vi "Get Vector - stdout.vi"(6 "no transpose\nfor reading":bool, 8 "error in (no error)":errorcluster, 9 "octave vector sizes":i32[](array[numeric]), 10 "variable name":string, 11 "pipe in":T1) -> (0 "error out":errorcluster, 2 "vector":string[](array[string]), 3 "pipe out":T1, 4 "value transposed?":bool)   [LabVIEW 2013, in "GOLPI library.lvlib"]
doc: "Reads vector variable from GNU Octave. Returns output as array of strings. Internaly converts row vector to column for simpler parsing of long vectors. It means complex vectors are conjugated and strings are incorrectly parsed. If 'no transpose for reading' is set true, function reads row vectors as rows."
uses:
  GOLPI library.lvlib
  LV Process.lvlibp/Pipe Handle.ctl
  Custom Error Codes Enum Type Def.vi
  Globals.vi
  LV Process.lvlibp
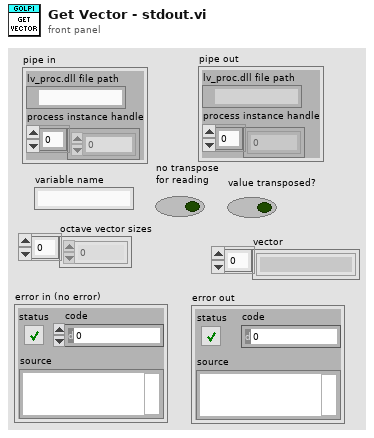
[diagram p1: front panel]
types:
  T1 = typedef "LV Process.lvlibp/Pipe Handle.ctl" = cluster{"lv_proc.dll file path":path, "process instance handle":u32[]}
  T2 = typedef "GOLPI library.lvlib/Custom Error Codes Enum Type Def.vi" = enum16{"no error", "00 working directory PAR1 missing", "01 octave binary PAR1 missing", "02 octave report error PAR1", "03 empty output last cmd PAR1", "04 missing temporary file PAR1", "10 var PAR1 not string", "11 var PAR1 not num, scal, ~compl", "12 var PAR1 not num, scal, compl", "13 var PAR1 not num, vect, ~compl", "14 var PAR1 not num, vect, compl", "15 var PAR1 not num, mat, ~compl", "16 var PAR1 not num, mat, ~compl", "99 not finished"}
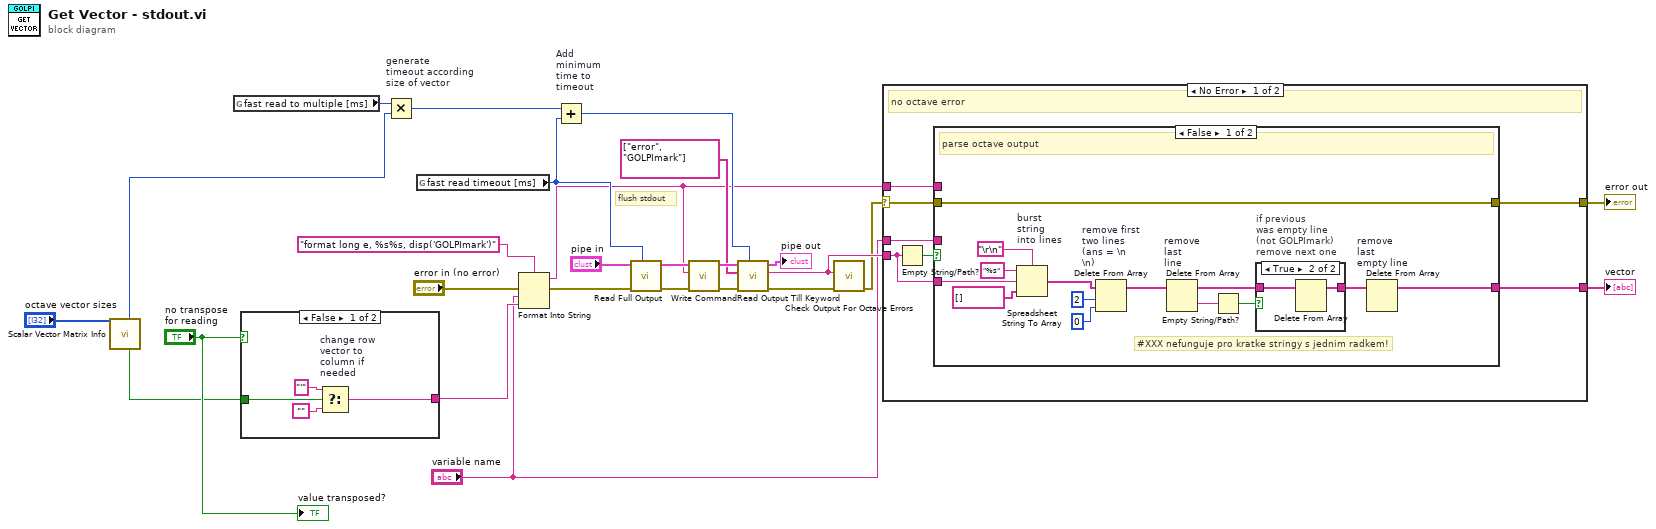
[diagram p0: block diagram]
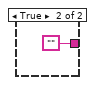
[diagram p2: hidden frame]
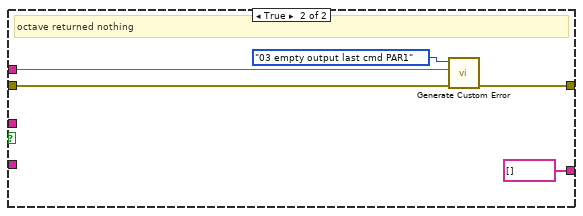
[diagram p4: hidden frame]
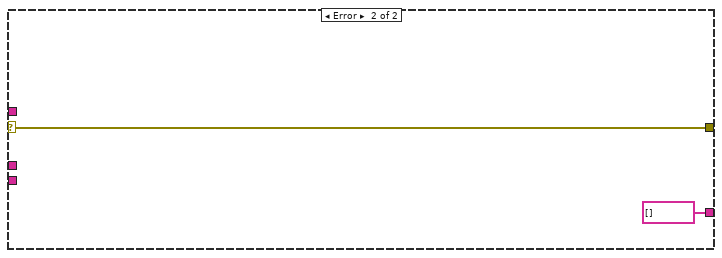
[diagram p5: hidden frame]
diagram:
  # "flush stdout"
  n1 = call "Scalar Vector Matrix Info.vi"("octave sizes"="octave vector sizes") -> ("row vector?"=w2:bool, "vector length"=w1:i32)  [unwired: 5 in, 4 out]
  n2 = global read "Globals.vi" "fast read to multiple [ms]"() -> (w11:u32)
  n3 = case shown="False" "no transpose\nfor reading" {
    tunnel: [w28 ""] -> w22
    tunnel: w2 -> [w27 _]
    frame False {
      n4 = Select "change row\nvector to\ncolumn if\nneeded"(t="'", s=w27, f="") -> (s? t:f=w28:string)
    }
    frame True {
    }
  }
  n5 = Multiply "generate\ntimeout according\nsize of vector"(x=w11, y=w1) -> (x*y=w18:u32)
  n6 = global read "Globals.vi" "fast read timeout [ms]"() -> (w12:u32)
  n7 = Format Into String(format string="format long e, %s%s, disp('GOLPImark')", error in="error in (no error)", "variable name", w22) -> (resulting string=w5:string, error out=w13:errorcluster)  [unwired: 1 in]
  n8 = Add "Add\nminimum\ntime to\ntimeout"(x=w18, y=w12) -> (x+y=w17:u32)
  n9 = call "Read Full Output.vi"("timeout [ms]"=w12, "error in"=w13, "pipe in"="pipe in") -> ("error out"=w14:errorcluster, "pipe out"=w15:T1)  [unwired: 5 in, 2 out]
  n10 = call "Write Command.vi"("error in"=w14, "command"=w5, "pipe in"=w15) -> ("error out"=w19:errorcluster, "pipe out"=w24:T1)  [unwired: 7 in]
  n11 = call "Read Output Till Keyword.vi"("timeout [ms]"=w17, "error in"=w19, "keywords"=string[] ["error", "GOLPImark"], "pipe in"=w24) -> ("error out"=w26:errorcluster, "read buffer"=w10:string, "pipe out"=→"pipe out":T1)  [unwired: 4 in, 1 out]
  n12 = call "Check Output For Octave Errors.vi"("error in"=w26, "read buffer"=w10) -> ("error out"=w6:errorcluster)  [unwired: 9 in]
  n13 = case shown="No Error" w6 {
    selector: w6 -> [w35 w62]
    tunnel: w10 -> [w34 _]
    tunnel: "variable name" -> [w38 _]
    tunnel: [w37 string[] []] -> w8
    tunnel: [w36 w62] -> w7
    tunnel: w5 -> [w32 _]
    frame No Error {
      # "no octave error"
      n14 = Empty String/Path?(string/path=w34) -> (empty?=w33:bool)
      n15 = case shown="False" w33 {
        tunnel: w34 -> [w48 _]
        tunnel: w38 -> [_ _]
        tunnel: [w39 string[] []] -> w37
        tunnel: w35 -> [w52 w58]
        tunnel: [w52 w57] -> w36
        tunnel: w32 -> [_ w56]
        frame False {
          # "#XXX nefunguje pro kratke stringy s jednim radkem!"
          # "parse octave output"
          n16 = Spreadsheet String To Array "burst\nstring\ninto lines"(delimiter (Tab)="\r\n", format string="%s", spreadsheet string=w48, array type (2D Dbl)=string[] []) -> (array=w47:string[])
          n17 = Delete From Array "remove first\ntwo lines\n(ans = \\n\n\\n)"(array=w47, length=2, index=0) -> (array with subset deleted=w44:string[])  [unwired: 1 out]
          n18 = Delete From Array "remove\nlast\nline"(array=w44) -> (deleted portion=w43:string, array with subset deleted=w42:string[])  [unwired: 2 in]
          n19 = Empty String/Path?(string/path=w43) -> (empty?=w40:bool)
          n20 = case "if previous\nwas empty line\n(not GOLPImark)\nremove next one" shown="True" w40 {
            tunnel: w42 -> [w53 w55]
            tunnel: [w53 w54] -> w41
            frame False {
            }
            frame True {
              n21 = Delete From Array(array=w55) -> (array with subset deleted=w54:string[])  [unwired: 2 in, 1 out]
            }
          }
          n22 = Delete From Array "remove\nlast\nempty line"(array=w41) -> (array with subset deleted=w39:string[])  [unwired: 2 in, 1 out]
        }
        frame True {
          # "octave returned nothing"
          n23 = call "Generate Custom Error.vi"("error in"=w58, "PAR1"=w56, "Enum"=Custom_Error_Codes_Enum_Type_Def.vi."03 empty output last cmd PAR1") -> ("error out"=w57:errorcluster)  [unwired: 8 in]
        }
      }
    }
    frame Error {
    }
  }
  "error out" <- w7
  "vector" <- w8
  "value transposed?" <- "no transpose\nfor reading"
